vi "ReadTraceItems.vi"(8 "ErrorIn":errorcluster) -> (0 "ErrorOut":errorcluster, 1 "TraceItems":T1[](array[typedef]))   [LabVIEW 2018, in "TracerLibrary.lvlib" / "Tracer.lvclass"]
uses:
  Tracer.lvclass
  TraceItemDefinition.ctl
  protected/Tracer_ClassAttributes.vi
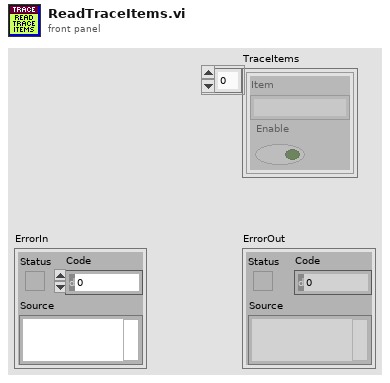
[diagram p1: front panel]
types:
  T1 = typedef "TracerLibrary.lvlib/Tracer.lvclass/TraceItemDefinition.ctl" = cluster{"Item":string, "Enable":bool}
  T2 = typedef "TRACE.lvlib/TRACE.lvclass/TRACE_ObjectAttributes.ctl" = cluster{"TraceContainer":variant}
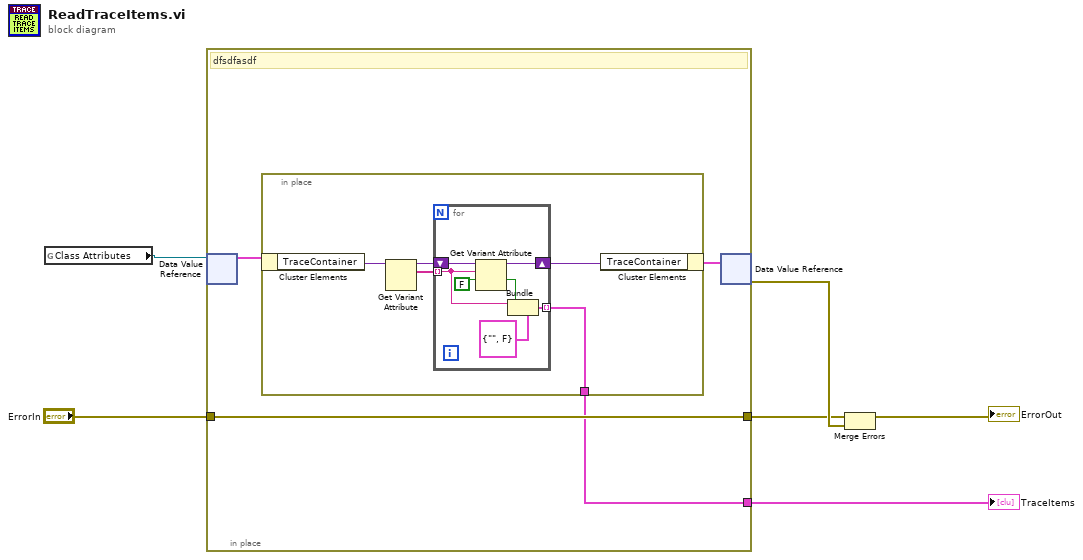
[diagram p0: block diagram]
diagram:
  n1 = global read "Tracer_ClassAttributes.vi" "Class Attributes"() -> (w2:refnum<data-value>)
  n2 = in-place {
    in-place-border: "ErrorIn" -> [w10]
    in-place-border: [w10] -> w3
    in-place-border: [w8] -> w1
    # "dfsdfasdf"
    n3 = in-place-dvr #1(w2) -> (w9:T2)  [unwired: 1 out]
    n4 = in-place {
      in-place-border: [w11] -> w8
      n5 = in-place-cluster #2(w9) -> ("TraceContainer"=w15:variant)
      n6 = Get Variant Attribute(Variant=w15) -> (duplicate Variant=w13:variant, names=w14:string[])  [unwired: 3 in, 2 out]
      n7 = for {
        tunnel: w14 -> [w18] mode=indexing
        shift-right: [w21] -> w12
        shift-left: w13 -> [w22]
        tunnel: [w16] -> w11 mode=indexing
        n8 = Get Variant Attribute(Variant=w22, name=w18, default value (empty Variant)=FALSE) -> (duplicate Variant=w21:variant, value=w17:bool)  [unwired: 1 in, 2 out]
        n9 = Bundle(cluster=T1 {"Item"="", "Enable"=FALSE} ("TraceItems"), "Item"=w18, "Enable"=w17) -> (w16:T1)
      }
      n10 = in-place-cluster #2("TraceContainer"=w12) -> (w7:T2)
    }
    n11 = in-place-dvr #1(w7) -> (w6:errorcluster)  [unwired: 1 out]
  }
  "TraceItems" <- w1
  n12 = Merge Errors(w3, w6) -> (→"ErrorOut":errorcluster)
